vi "UI.Set.vi"(10 "data value":T1, 11 "DVR.state":T2) -> ()   [LabVIEW 2020]
uses:
  _controls/data.ctl
  camera/camera.lvclass
  _controls/data.ref.ctl
  <vilib>/vision/Image Controls.llb/IMAQ Image.ctl
  _controls/state.ctl
  _controls/data.vars.ctl
  _controls/flip.ctl
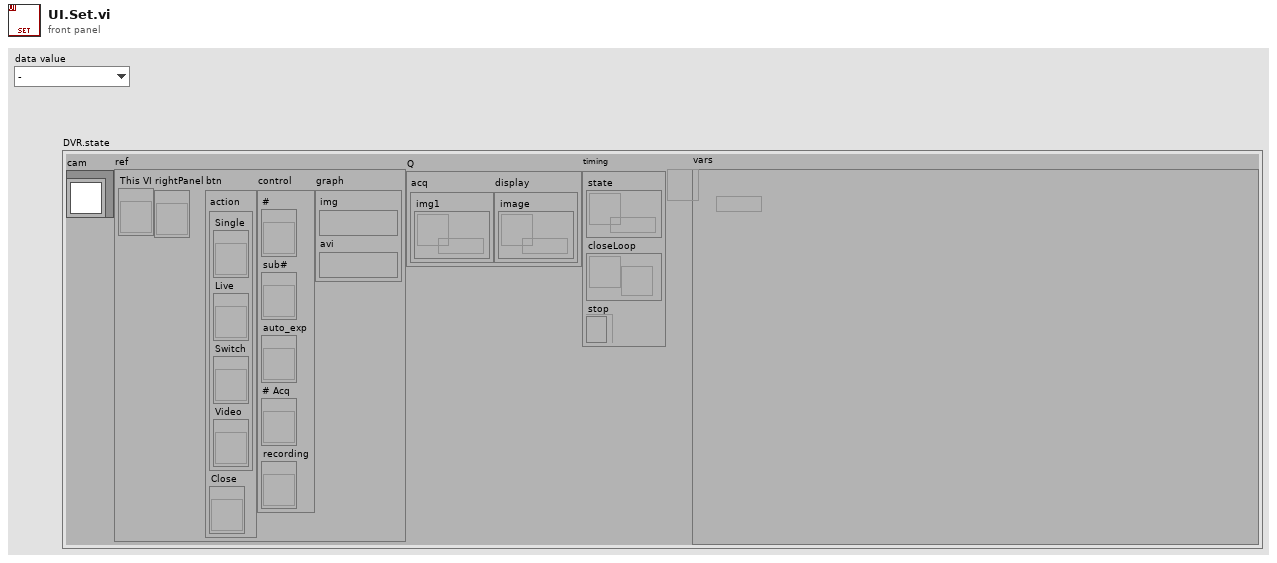
[diagram p1: front panel]
types:
  T1 = typedef "state.ctl" = enum16{"-", "single", "video", "livePL", "PL"}
  T2 = typedef "data.ctl" = cluster{"cam":refnum<class "camera.lvclass">, "ref":T3, "Q":cluster{"acq":cluster{"img1":refnum<queue>}, "display":cluster{"image":refnum<queue>}}, "timing":cluster{"state":refnum<queue>, "closeLoop":refnum<notifier>, "stop":refnum<k4>}, "vars":refnum<data-value>}
  T3 = typedef "data.ref.ctl" = cluster{"This VI":refnum<vi>, "rightPanel":refnum<vi>, "btn":cluster{"action":cluster{"Single":refnum<vi>, "Live":refnum<vi>, "Switch":refnum<vi>, "Video":refnum<vi>}, "Close":refnum<vi>}, "control":cluster{"#":refnum<vi>, "sub#":refnum<vi>, "auto_exp":refnum<vi>, "# Acq":refnum<vi>, "recording":refnum<vi>}, "graph":cluster{"img":T4, "avi":T4}}
  T4 = typedef "IMAQ Image.ctl" = refnum<image>
  T5 = enum8{"Enabled", "Disabled", "Disabled and Grayed Out"}
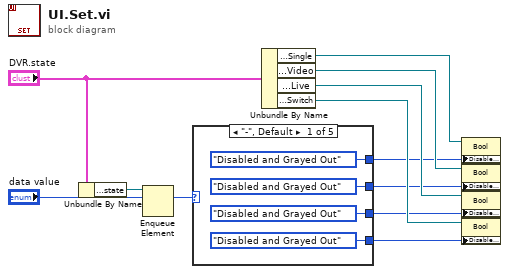
[diagram p0: block diagram]
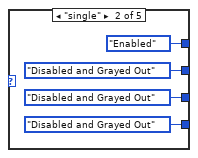
[diagram p2: hidden frame]
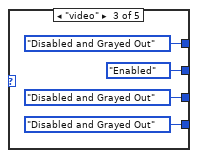
[diagram p3: hidden frame]
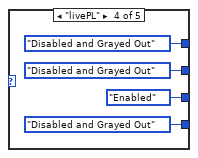
[diagram p4: hidden frame]
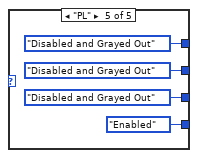
[diagram p5: hidden frame]
diagram:
  n1 = Unbundle By Name("DVR.state") -> ("timing.state"=w2:refnum<queue>)
  n2 = Enqueue Element(queue=w2, element="data value") -> ()  [unwired: 2 in, 3 out]
  n3 = case shown="\"-\", Default" "data value" {
    tunnel: [T5."Disabled and Grayed Out" ("Disabled") T5."Enabled" ("Disabled") T5."Disabled and Grayed Out" ("Disabled") T5."Disabled and Grayed Out" ("Disabled") T5."Disabled and Grayed Out" ("Disabled")] -> w7
    tunnel: [T5."Disabled and Grayed Out" ("Disabled") T5."Disabled and Grayed Out" ("Disabled") T5."Enabled" ("Disabled") T5."Disabled and Grayed Out" ("Disabled") T5."Disabled and Grayed Out" ("Disabled")] -> w6
    tunnel: [T5."Disabled and Grayed Out" ("Disabled") T5."Disabled and Grayed Out" ("Disabled") T5."Disabled and Grayed Out" ("Disabled") T5."Enabled" ("Disabled") T5."Disabled and Grayed Out" ("Disabled")] -> w5
    tunnel: [T5."Disabled and Grayed Out" ("Disabled") T5."Disabled and Grayed Out" ("Disabled") T5."Disabled and Grayed Out" ("Disabled") T5."Disabled and Grayed Out" ("Disabled") T5."Enabled" ("Disabled")] -> w4
    frame "-", Default {
    }
    frame "single" {
    }
    frame "video" {
    }
    frame "livePL" {
    }
    frame "PL" {
    }
  }
  n4 = Unbundle By Name("DVR.state") -> ("ref.btn.action.Single"=w8:refnum<vi>, "ref.btn.action.Video"=w9:refnum<vi>, "ref.btn.action.Live"=w10:refnum<vi>, "ref.btn.action.Switch"=w11:refnum<vi>)
  n5 = property class="Bool"(reference=w8, "DisabledEnum"=w7) -> ()  [unwired: 1 in, 2 out]
  n6 = property class="Bool"(reference=w9, "DisabledEnum"=w6) -> ()  [unwired: 1 in, 2 out]
  n7 = property class="Bool"(reference=w10, "DisabledEnum"=w5) -> ()  [unwired: 1 in, 2 out]
  n8 = property class="Bool"(reference=w11, "DisabledEnum"=w4) -> ()  [unwired: 1 in, 2 out]
